vi "BallAtDefenseAreaGoalie.vi"(9 "Field defense":dbl[](array[numeric]), 10 "IA State":T1={"our_robots"=[], "enemy_robots"=[], "balls"=[], "geometry"={"line_width"=0, "field_length"=0, "field_width"=0, "boundary_width"=0, "referee_width"=0, "goal_width"=0, "goal_depth"=0, "goal_wall_width"=0, "center_circle_radius"=0, "defense_radius"=0, "defense_stretch"=0, "free_kick_from_defense_dist"=0, "penalty_spot_from_field_line_dist"=0, "penalty_line_from_spot_dist"=0}, "IA Judge"={"stage"="", "command"="", "our_goalie_id"=0.0, "enemy_goalie_id"=0.0, "command enum"=enum."Halt", "Time"=enum."Azul"}, "Received Timestamp"=timestamp(0 s since 1904-01-01), "Events"={"Touch"=FALSE, "Ball out"=FALSE, "id touch"=0.0, "Ball out of \nVision"=FALSE, "Ball inside \nGoalie area"=FALSE, "Robot not responding"=FALSE, "Robots responding status"=[1.0, 1.0, 1.0, 1.0, 1.0, 1.0], "Enemy Ball \nPossession"=FALSE, "Pass State"=FALSE, "id end of pass"=0.0, "Kick"=FALSE, "Id ini Possession"=0.0, "Ball Possesion"=FALSE, "Id Possesion"=0.0}}) -> (2 "Ball at goalkeeper area ?":bool)   [LabVIEW 2016]
uses:
  Core/AI Input.ctl
  Core/AI Robot.ctl
  Intel/Functions Enum.ctl
  Intel/AttackerStates.ctl
  Core/AI Ball.ctl
  Core/Field Size.ctl
  Core/AI Judge.ctl
  Intel/Command Enum.ctl
  Events/Events.ctl
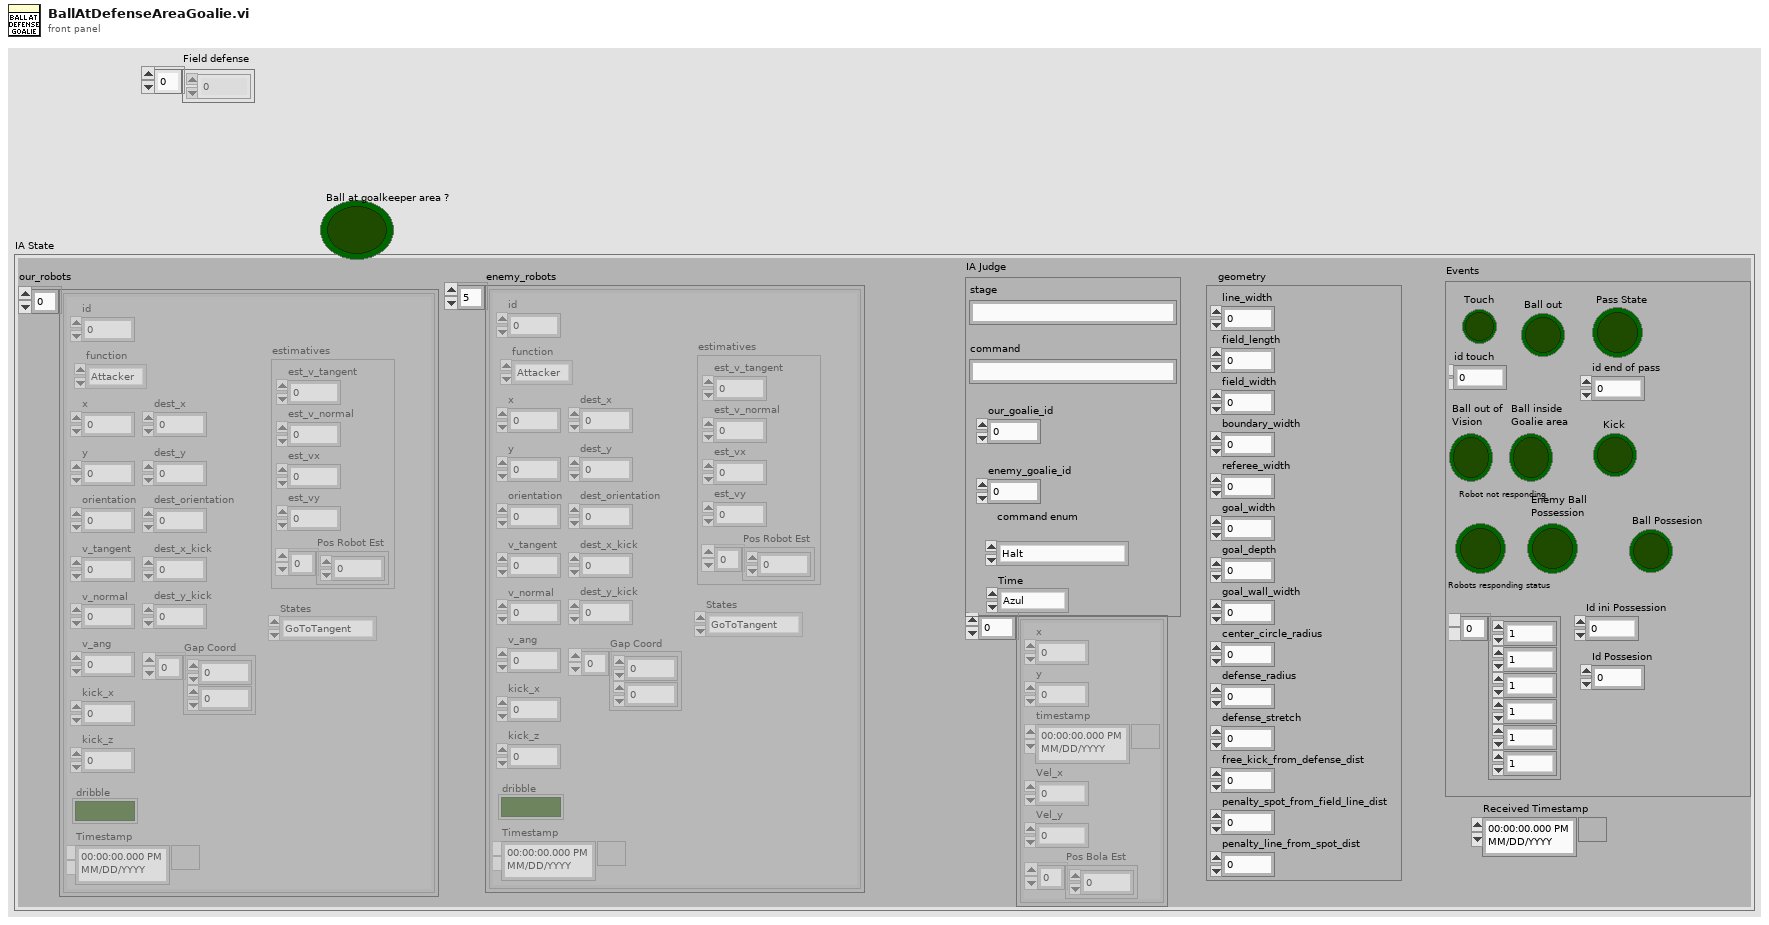
[diagram p1: front panel]
types:
  T1 = typedef "AI Input.ctl" = cluster{"our_robots":T2[], "enemy_robots":T2[], "balls":T5[], "geometry":T6, "IA Judge":T7, "Received Timestamp":timestamp, "Events":T9}
  T2 = typedef "AI Robot.ctl" = cluster{"id":u32, "function":T3, "x":dbl, "y":dbl, "orientation":dbl, "v_tangent":dbl, "v_normal":dbl, "v_ang":dbl, "kick_x":dbl, "kick_z":dbl, "dribble":bool, "Timestamp":timestamp, "dest_x":dbl, "dest_y":dbl, "dest_orientation":dbl, "estimatives":cluster{"est_v_tangent":dbl, "est_v_normal":dbl, "est_vx":dbl, "est_vy":dbl, "Pos Robot Est":dbl[]}, "dest_x_kick":dbl, "dest_y_kick":dbl, "Gap Coord":dbl[], "States":T4}
  T3 = typedef "Functions Enum.ctl" = enum16{"Attacker", "Goalie", "Defender", "Striker", "Goto 0", "Dummy", "Kicker", "ZigZag"}
  T4 = typedef "AttackerStates.ctl" = enum16{"Pass", "GoToTangent", "BallGetting", "GoToKick", ""}
  T5 = typedef "AI Ball.ctl" = cluster{"x":dbl, "y":dbl, "timestamp":timestamp, "Vel_x":dbl, "Vel_y":dbl, "Pos Bola Est":dbl[]}
  T6 = typedef "Field Size.ctl" = cluster{"line_width":u32, "field_length":u32, "field_width":u32, "boundary_width":u32, "referee_width":u32, "goal_width":u32, "goal_depth":u32, "goal_wall_width":u32, "center_circle_radius":u32, "defense_radius":u32, "defense_stretch":u32, "free_kick_from_defense_dist":u32, "penalty_spot_from_field_line_dist":u32, "penalty_line_from_spot_dist":u32}
  T7 = typedef "AI Judge.ctl" = cluster{"stage":string, "command":string, "our_goalie_id":dbl, "enemy_goalie_id":dbl, "command enum":T8, "Time":enum16{"Azul", "Amarelo"}}
  T8 = typedef "Command Enum.ctl" = enum16{"Halt", "Stop", "Force Start", "PKA Normal Start", "Prepare Kickoff Ally", "PKE Normal Start", "Prepare Kickoff Enemy", "Prepare Penalty Ally", "PPA Normal Start", "Prepare Penalty Enemy", "PPE Normal Start", "Direct Free Enemy", "Direct Free Ally", "Indirect Free Enemy", "Indirect Free Ally", "Timeout Enemy", "Timeout Ally", "Goal Enemy", "Goal Ally", "Ball Placement Enemy", "Ball Placement Ally", "Normal Half Time", "Extra Time Break", "Extra Half Time", "None", "Post Game"}
  T9 = typedef "Events.ctl" = cluster{"Touch":bool, "Ball out":bool, "id touch":dbl, "Ball out of \nVision":bool, "Ball inside \nGoalie area":bool, "Robot not responding":bool, "Robots responding status":dbl[], "Enemy Ball \nPossession":bool, "Pass State":bool, "id end of pass":dbl, "Kick":bool, "Id ini Possession":dbl, "Ball Possesion":bool, "Id Possesion":dbl}
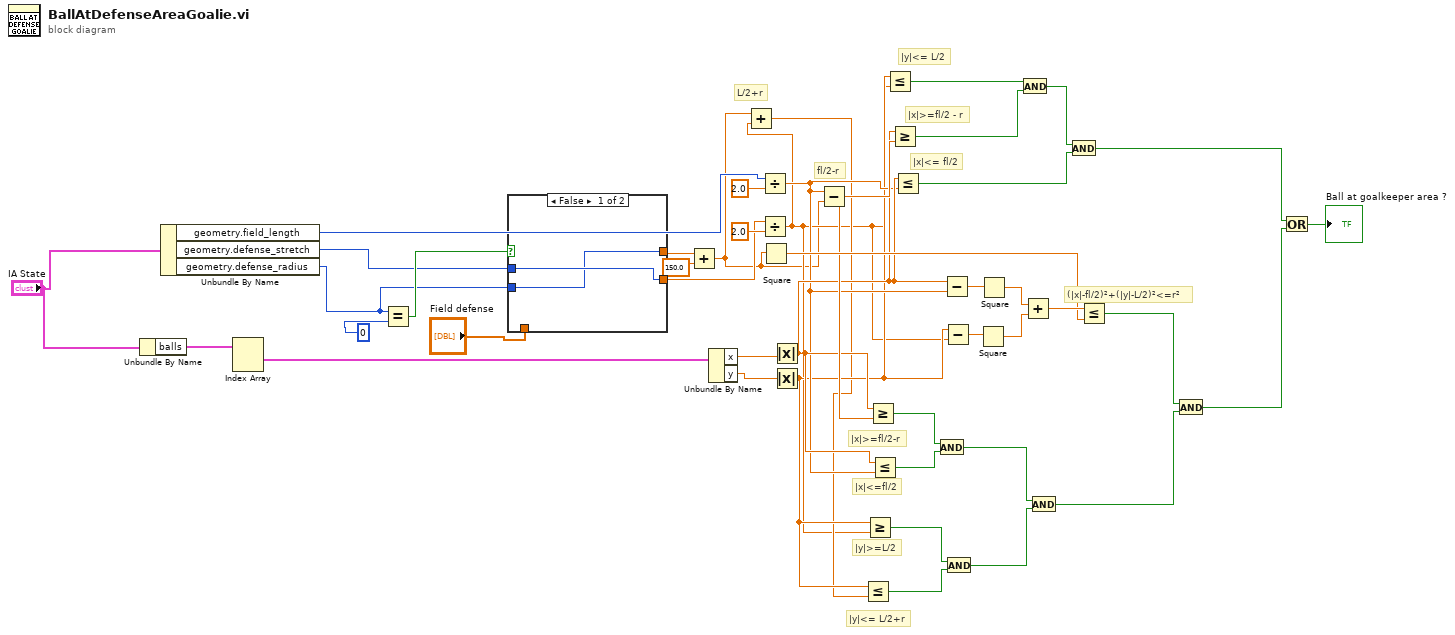
[diagram p0: block diagram]
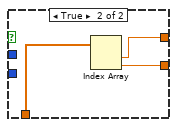
[diagram p2: hidden frame]
diagram:
  # "|y|<= L/2+r"
  # "L/2+r"
  # "|y|>=L/2"
  # "|x|<=fl/2"
  # "|x|>=fl/2-r"
  # "fl/2-r"
  # "(|x|-fl/2)²+(|y|-L/2)²<=r²"
  # "|x|<= fl/2"
  # "|x|>=fl/2 - r"
  # "|y|<= L/2"
  n1 = Unbundle By Name("IA State") -> ("balls"=w44:T5[])
  n2 = Unbundle By Name("IA State") -> ("geometry.field_length"=w37:u32, "geometry.defense_stretch"=w5:u32, "geometry.defense_radius"=w4:u32)
  n3 = Index Array(array=w44) -> (element #1=w43:T5)  [unwired: 2 in, 1 out]
  n4 = Equal?(x=w4, y=u32 0) -> (x = y?=w7:bool)
  n5 = case shown="False" w7 {
    tunnel: [w45 w49] -> w3
    tunnel: [w46 w48] -> w6
    tunnel: "Field defense" -> [_ w47]
    tunnel: w5 -> [w46 _]
    tunnel: w4 -> [w45 _]
    frame False {
    }
    frame True {
      n6 = Index Array(array=w47) -> (element #1=w49:dbl, element #2=w48:dbl)  [unwired: 2 in]
    }
  }
  n7 = Add(x=w3, y=150.0) -> (x+y=w2:dbl)
  n8 = Unbundle By Name(w43) -> ("x"=w40:dbl, "y"=w41:dbl)
  n9 = Divide(x=w37, y=2.0) -> (x/y=w22:dbl)
  n10 = Divide(x=w6, y=2.0) -> (x/y=w10:dbl)
  n11 = Add(x=w2, y=w10) -> (x+y=w20:dbl)
  n12 = Square(x=w2) -> (x^2=w27:dbl)
  n13 = Absolute Value(x=w40) -> (abs(x)=w25:dbl)
  n14 = Absolute Value(x=w41) -> (abs(x)=w21:dbl)
  n15 = Subtract(x=w22, y=w2) -> (x-y=w26:dbl)
  n16 = Less Or Equal?(x=w21, y=w20) -> (x <= y?=w18:bool)
  n17 = Greater Or Equal?(x=w21, y=w10) -> (x >= y?=w19:bool)
  n18 = Greater Or Equal?(x=w25, y=w26) -> (x >= y?=w24:bool)
  n19 = Less Or Equal?(x=w25, y=w22) -> (x <= y?=w23:bool)
  n20 = Less Or Equal?(x=w21, y=w10) -> (x <= y?=w36:bool)
  n21 = Greater Or Equal?(x=w25, y=w26) -> (x >= y?=w35:bool)
  n22 = Less Or Equal?(x=w25, y=w22) -> (x <= y?=w33:bool)
  n23 = And(x=w24, y=w23) -> (x .and. y?=w17:bool)
  n24 = Subtract(x=w25, y=w22) -> (x-y=w32:dbl)
  n25 = Subtract(x=w21, y=w10) -> (x-y=w31:dbl)
  n26 = And(x=w19, y=w18) -> (x .and. y?=w16:bool)
  n27 = Square(x=w31) -> (x^2=w29:dbl)
  n28 = Square(x=w32) -> (x^2=w30:dbl)
  n29 = And(x=w36, y=w35) -> (x .and. y?=w34:bool)
  n30 = Add(x=w30, y=w29) -> (x+y=w28:dbl)
  n31 = And(x=w17, y=w16) -> (x .and. y?=w14:bool)
  n32 = And(x=w34, y=w33) -> (x .and. y?=w13:bool)
  n33 = Less Or Equal?(x=w28, y=w27) -> (x <= y?=w15:bool)
  n34 = And(x=w15, y=w14) -> (x .and. y?=w12:bool)
  n35 = Or(x=w13, y=w12) -> (x .or. y?=→"Ball at goalkeeper area ?":bool)
